vi "SR830-MinimalNoiseSetup.vi"(0 "VISA resource name":refnum<visa-resource-name>="SR830LockIn2", 5 "Rl":dbl=24060.0 format="%#_13g", 7 "number of averaging points":i32=10, 9 "Rp":dbl=1010.0 format="%#_13g", 11 "error in (no error)":errorcluster) -> (1 "Vs (Vrms)":dbl, 3 "Time Constant (s)":dbl, 4 "VISA resource name out":refnum<visa-resource-name>, 6 "Wait Time (s)":dbl, 8 "ENBW":dbl, 10 "Number of samples Averaged":dbl, 12 "Filter slope (dB/oct)":dbl, 14 "Setup Data":T1, 15 "error out":errorcluster)   [LabVIEW 2016]
panel:
  # "This VI sets up the number of samples to average based off of the filter slope, time constant, and measurment time.\nIt also outputs the time constant and the stabilizing wait time for proper measurements.\nIf the R-stdev or Theta-stdev are too large, adjust settings on the SR830 before continuing."
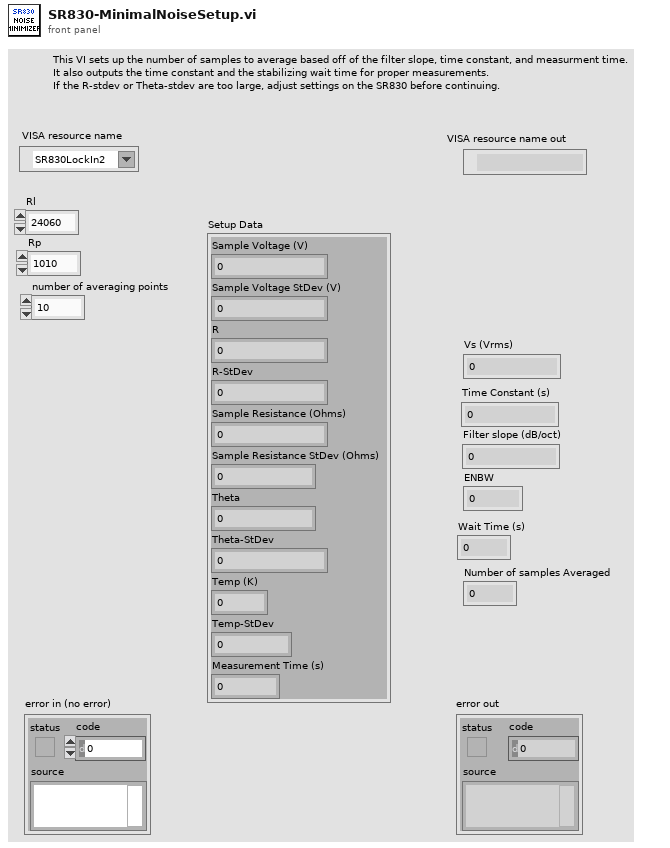
[diagram p1: front panel]
types:
  T1 = cluster{"Sample Voltage (V)":dbl, "Sample Voltage StDev (V)":dbl, "R":dbl, "R-StDev":dbl, "Sample Resistance (Ohms)":dbl, "Sample Resistance StDev (Ohms)":dbl, "Theta":dbl, "Theta-StDev":dbl, "Temp (K)":dbl, "Temp-StDev":dbl, "Measurement Time (s)":dbl}
  T2 = cluster{"Sample Voltage (V)":dbl, "Sample Voltage StDev (V)":dbl, "R":dbl, "R-StDev":dbl, "Sample Resistance (Ohms)":dbl, "Sample Resistance StDev (Ohms)":dbl, "Theta (degrees)":dbl, "Theta-StDev (degrees)":dbl, "Temp (K)":dbl, "Temp-StDev":dbl, "Measurement Time (s)":dbl}
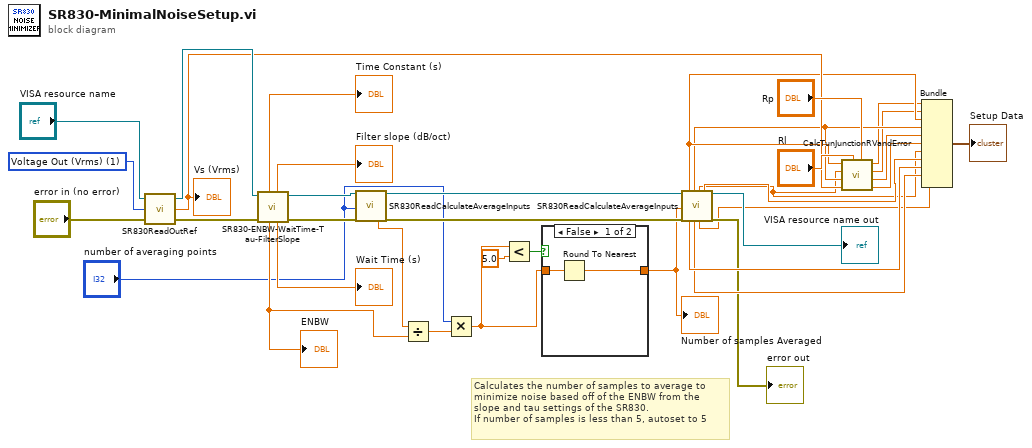
[diagram p0: block diagram]
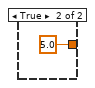
[diagram p2: hidden frame]
diagram:
  w17 = u16 1 items=["Voltage Out (Vrms)"=1, "Frequency (Hz)"=2, "Aux Out 1 (VDC)"=3, "Aux Out 2 (VDC)"=4, "Time Constant (s)"=5, "Roll-Off Slope (dB/oct)"=6] ("ReadOut (1: Voltage Amplitude)")
  # "Calculates the number of samples to average to \nminimize noise based off of the ENBW from the \nslope and tau settings of the SR830.\nIf number of samples is less than 5, autoset to 5"
  n1 = call "SR830ReadOutRef.vi"("error in (no error)"="error in (no error)", "ReadOut (1: Voltage Amplitude)"=w17, "VISA resource name"="VISA resource name") -> ("error out"=w15:errorcluster, "ReadOut"=w11:dbl, "VISA resource name out"=w16:refnum<visa-resource-name>)
  "Vs (Vrms)" <- w11
  n2 = call "SR830-ENBW-WaitTime-Tau-FilterSlope.vi"("error in (no error)"=w15, "VISA resource name"=w16) -> ("error out"=w36:errorcluster, "VISA resource name out"=w37:refnum<visa-resource-name>, "Wait Time (s)"=→"Wait Time (s)":dbl, "Filter slope (dB/oct)"=→"Filter slope (dB/oct)":dbl, "ENBW"=w35:dbl, "Time Constant (s)"=→"Time Constant (s)":dbl)  [unwired: 4 in]
  "ENBW" <- w35
  n3 = call "SR830ReadCalculateAverageInputs.vi"("VISA resource name"=w37, "number of averaging points"="number of averaging points", "error in (no error)"=w36) -> ("Measurement Bandwidth (Hz)"=w2:dbl, "VISA resource name out"=w30:refnum<visa-resource-name>, "error out"=w29:errorcluster)  [unwired: 7 in, 7 out]
  n4 = Divide(x=w2, y=w35) -> (x/y=w34:dbl)
  n5 = Multiply(x="number of averaging points", y=w34) -> (x*y=w31:dbl)
  n6 = Less?(x=w31, y=5.0) -> (x < y?=w32:bool)
  n7 = case shown="False" w32 {
    tunnel: w31 -> [w39 _]
    tunnel: [w38 5.0 ("y")] -> w28
    frame False {
      n8 = Round To Nearest(number=w39) -> (nearest integer value=w38:dbl)
    }
    frame True {
    }
  }
  "Number of samples Averaged" <- w28
  n9 = call "SR830ReadCalculateAverageInputs.vi"("VISA resource name"=w30, "number of averaging points"=w28, "error in (no error)"=w29) -> ("R"=w10:dbl, "Temp (K)"=w26:dbl, "R-StDev"=w9:dbl, "Temp-StDev"=w25:dbl, "Theta (degrees)"=w8:dbl, "Measurement Time (s)"=w1:dbl, "Theta-StDev (degrees)"=w27:dbl, "VISA resource name out"=→"VISA resource name out":refnum<visa-resource-name>, "error out"=→"error out":errorcluster)  [unwired: 7 in, 1 out]
  n10 = call "CalcTunJunctionRVandError.vi"("Rp"="Rp", "Rl"="Rl", "Source Voltage (V)"=w11, "Sample Current StDev (A)"=w9, "Sample Current Theta (degrees)"=w8, "Sample Current R (A)"=w10) -> ("Sample Resistance StDev (Ohms)"=w4:dbl, "Sample Resistance (Ohms)"=w5:dbl, "Sample Voltage StDev (V)"=w6:dbl, "Sample Voltage (V)"=w7:dbl)  [unwired: 2 in]
  n11 = Bundle("Sample Voltage (V)"=w7, "Sample Voltage StDev (V)"=w6, "R"=w10, "R-StDev"=w9, "Sample Resistance (Ohms)"=w5, "Sample Resistance StDev (Ohms)"=w4, "Theta (degrees)"=w8, "Theta-StDev (degrees)"=w27, "Temp (K)"=w26, "Temp-StDev"=w25, "Measurement Time (s)"=w1) -> (→"Setup Data":T2)  [unwired: 1 in]
